vi "Formula_Node_Ejercicio.vi"() -> ()   [LabVIEW 2020]
panel:
  out "XY Graph":cluster{dbl[], dbl[]}(graph)
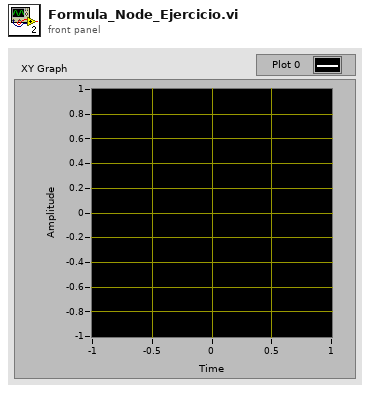
[diagram p1: front panel]
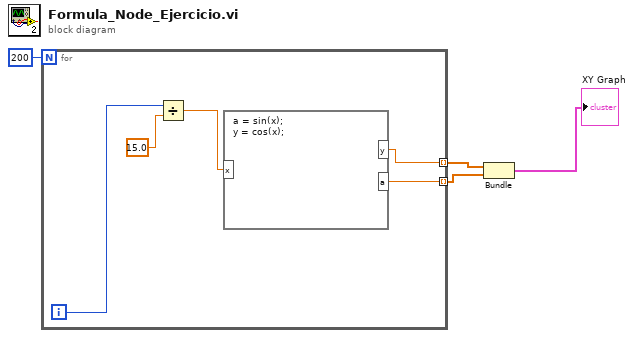
[diagram p0: block diagram]
diagram:
  n1 = for {
    N: 200 -> [_]
    tunnel: [w6] -> w3 mode=indexing
    tunnel: [w5] -> w2 mode=indexing
    i -> [w9]
    n2 = Divide(x=w9, y=15.0) -> (x/y=w7:dbl)
    n3 = formula code="a = sin(x);\ny = cos(x);"("x"=w7) -> ("y"=w6:dbl, "a"=w5:dbl)
  }
  n4 = Bundle(w3, w2) -> (→"XY Graph":cluster{dbl[], dbl[]})  [unwired: 1 in]
